vi "Autonomous Independent.vi"() -> ()   [LabVIEW 2014]
doc: "This VI is called when autonomous begins, and will automatically be terminated when autonomous ends. You can carry out timed or sensor driven robot movement independently without needing to return to the caller."
uses:
  <vilib>/Rock Robotics/Network Tables/SD Write Numeric Array.vi
  <vilib>/addons/control/pid/NI_PID_pid.lvlib
  <vilib>/addons/control/pid/pid.llb/PID (DBL).vi
  Robot Global Data.vi
  <vilib>/Rock Robotics/WPI/RobotDrive/WPI_RobotDriveMotorSelectorEnum.ctl
  <vilib>/Rock Robotics/WPI/CAN/TalonSRX/WPI_CANTalonSRX_APIControlMode.ctl
panel:
  in  "(Left) First Step":dbl
  in  "(Right) First Step":dbl
  in  "Left Wheel Distance":dbl
  in  "Right Wheel Distance":dbl
  in  "(Right) First Step":dbl
  in  "(Left) First Step":dbl
  # "Be sure to right-click and choose Data Operations>>Make Current Value default if you want to save the array values with the VI"
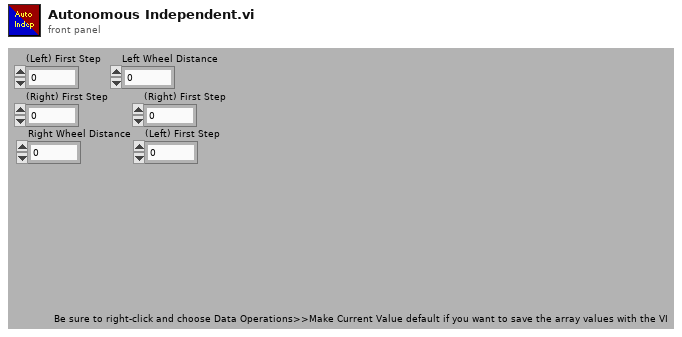
[diagram p1: front panel]
types:
  T1 = typedef "WPI_CANTalonSRX_APIControlMode.ctl" = enum8{"Percent VBus", "Speed", "Position", "Slave", "Unchanged / Invalid"}
  T2 = typedef "WPI_RobotDriveMotorSelectorEnum.ctl" = enum16{"Rear Left Motor", "Rear Right Motor", "Front Left Motor", "Front Right Motor"}
  T3 = typedef "WPI_JoystickDevRef.ctl" = cluster{"Device":T4}
  T4 = typedef "WPI_JoystickDeviceEnum.ctl" = enum16{"USB 0", "USB 1", "USB 2", "USB 3", "USB 4", "USB 5"}
  T5 = typedef "WPI_RobotDriveDevRef.ctl" = cluster{"DevStatus":errorcluster, "Motors[]":T6[], "Square Inputs":bool, "Max Output":dbl}
  T6 = typedef "WPI_MotorControlDeviceRef.ctl" = cluster{"DeviceStatus":errorcluster, "Type":T7, "PWM":cluster{"Controller":T8, "PWM Channel":T9, "DeadBand":T10}, "CAN":cluster{"Device Number":u8, "Control Mode":T11, "Semaphore":T12, "Max Vout":dbl, "TalonSRX Control Mode":T1}, "Invert":bool, "TransformRef":T13, "InvTransformRef":T13}
  T7 = typedef "WPI_MotorControlType.ctl" = enum16{"PWM", "CAN", "CANTalonSRX"}
  T8 = typedef "FPGA_TypedefDigitalModule.ctl" = enum16{"Controller 1"}
  T9 = typedef "FPGA_DIOPWMChannel.ctl" = enum8{"PWM 0", "PWM 1", "PWM 2", "PWM 3", "PWM 4", "PWM 5", "PWM 6", "PWM 7", "PWM 8", "PWM 9", "PWM MXP 0", "PWM MXP 1", "PWM MXP 2", "PWM MXP 3", "PWM MXP 4", "PWM MXP 5", "PWM MXP 6", "PWM MXP 7", "PWM MXP 8", "PWM MXP 9", "Invalid"}
  T10 = typedef "WPI_PWMDeadband.ctl" = cluster{"Name":string, "maxPositivePwm":i32, "minPositivePwm":i32, "centerPwm":i32, "maxNegativePwm":i32, "minNegativePwm":i32, "angularRange":u16}
  T11 = typedef "WPI_CANJaguar_ControlMode.ctl" = enum8{"Percent VBus", "Current", "Speed", "Position", "Voltage"}
  T12 = typedef "Semaphore RefNum" = refnum<k1>
  T13 = typedef "WPI_PWMTransform_ConPane.ctl" = refnum<vi>
  T14 = typedef "WPI_SwitchDevRef.ctl" = cluster{"DevStatus":errorcluster, "DIO Channel":T15, "Controller":T8, "CntIndex":T16, "Normally Closed":bool}
  T15 = typedef "FPGA_DIOChannel.ctl" = enum8{"DIO 0", "DIO 1", "DIO 2", "DIO 3", "DIO 4", "DIO 5", "DIO 6", "DIO 7", "DIO 8", "DIO 9", "DIO MXP 0", "DIO MXP 1", "DIO MXP 2", "DIO MXP 3", "DIO MXP 4", "DIO MXP 5", "DIO MXP 6", "DIO MXP 7", "DIO MXP 8", "DIO MXP 9", "DIO MXP 10", "DIO MXP 11", "DIO MXP 12", "DIO MXP 13", "DIO MXP 14", "DIO MXP 15", "Invalid"}
  T16 = typedef "FPGA_CounterCtrSystemIndex.ctl" = enum8{"Ctr 0", "Ctr 1", "Ctr 2", "Ctr 3", "Ctr 4", "Ctr 5", "Ctr 6", "Ctr 7", "Invalid"}
  T17 = typedef "WPI_CANTalonSRX_GlobalStatus.ctl" = cluster{"Applied Throttle":dbl, "Module Enabled":bool, "CAN Error":errorcluster, "Closed Loop Error":dbl, "Forward Limit Switch Closed":bool, "Reverse Limit Switch Closed":bool, "Sensor Position":dbl, "Sensor Velocity":dbl, "Current":dbl, "Sticky Fault - Over Temp":bool, "Sticky Fault - Under Voltage":bool, "Sticky Fault - Forward Limit":bool, "Sticky Fault - Reverse Limit":bool, "Sticky Fault - Forward Soft Limit":bool, "Sticky Fault - Reverse Soft Limit":bool, "Brake is Enabled":bool, "Encoder Position":dbl, "Encoder Velocity":dbl, "Encoder Index Count":dbl, "Encoder A Pin State":bool, "Encoder B Pin State":bool, "Encoder Index Pin State":bool, "Analog In":dbl, "Analog In Velocity":dbl, "Temperature (C)":dbl, "Battery Voltage":dbl}
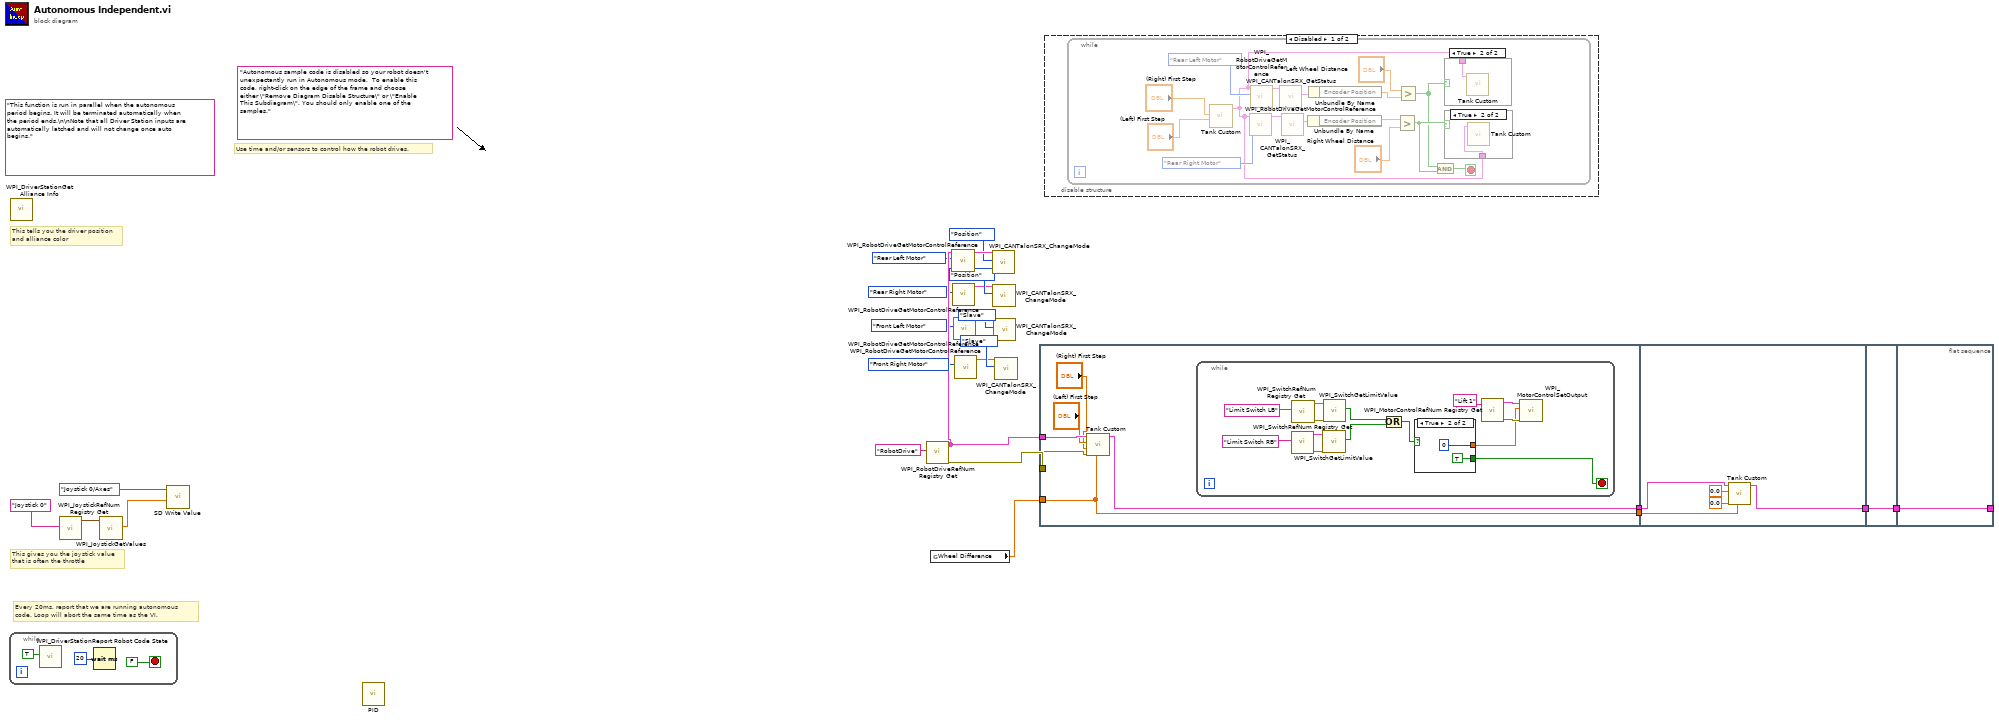
[diagram p0: block diagram]
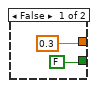
[diagram p5: hidden frame]
diagram:
  (unwired) "Autonomous sample code is disabled so your robot doesn't unexpectantly run in Autonomous mode.  To enable this code, right-click on the edge of the frame and choose either \"Remove Diagram Disable Structure\" or \"Enable This Subdiagram\". You should only enable one of the samples."
  (unwired) "This function is run in parallel when the autonomous period begins. It will be terminated automatically when the period ends.\n\nNote that all Driver Station inputs are automatically latched and will not change once auto begins."
  # "Every 20ms, report that we are running autonomous\ncode. Loop will abort the same time as the VI."
  # "This gives you the joystick value\nthat is often the throttle"
  # "Use time and/or sensors to control how the robot drives."
  # "This tells you the driver position\nand alliance color"
  n1 = while {
    stop <- FALSE stop-if-true
    n2 = call <vilib>:"WPI_DriverStationReport Robot Code State.vi"("Autonomous"=TRUE) -> ()  [unwired: 10 in, 1 out]
    n3 = Wait (ms)(milliseconds to wait=u32 20) -> ()  [unwired: 1 out]
  }
  n4 = call <vilib>:"WPI_DriverStationGet Alliance Info.vi"() -> ()  [unwired: 12 out]
  n5 = call <vilib>:"WPI_JoystickRefNum Registry Get.vi"("refnum name"="Joystick 0") -> ("JoystickDevRef"=w23:T3)  [unwired: 1 in, 9 out]
  n6 = call <vilib>:"WPI_JoystickGetValues.vi"("JoystickDevRef"=w23) -> ("Axes"=w21:dbl[])  [unwired: 6 in, 4 out]
  n7 = call-poly <vilib>:"SD Write Value.vi"("Numeric Array"=w21, "Name"="Joystick 0/Axes") -> ()  [unwired: 8 in, 2 out]
  n8 = call-poly <vilib>:"PID.vi"() -> ()  [unwired: 10 in, 2 out]
  n9 = call <vilib>:"WPI_RobotDriveRefNum Registry Get.vi"("refnum name"="RobotDrive") -> ("error out"=w15:errorcluster, "RobotDriveDevRef"=w12:T5)  [unwired: 1 in, 8 out]
  n10 = global read "Robot Global Data.vi" "Wheel Difference"() -> (w14:dbl)
  n11 = call <vilib>:"WPI_RobotDriveGetMotorControlReference.vi"("MotorIndex"=WPI_RobotDriveMotorSelectorEnum."Rear Left Motor", "RobotDriveDevRef"=w12) -> ("MotorControlDeviceRef"=w13:T6)  [unwired: 9 out]
  n12 = call <vilib>:"WPI_RobotDriveGetMotorControlReference.vi"("MotorIndex"=WPI_RobotDriveMotorSelectorEnum."Rear Right Motor") -> ("MotorControlDeviceRef"=w7:T6)  [unwired: 1 in, 9 out]
  n13 = call <vilib>:"WPI_RobotDriveGetMotorControlReference.vi"("MotorIndex"=WPI_RobotDriveMotorSelectorEnum."Front Left Motor") -> ("MotorControlDeviceRef"=w6:T6)  [unwired: 1 in, 9 out]
  n14 = call <vilib>:"WPI_RobotDriveGetMotorControlReference.vi"("MotorIndex"=WPI_RobotDriveMotorSelectorEnum."Front Right Motor") -> ("MotorControlDeviceRef"=w1:T6)  [unwired: 1 in, 9 out]
  n15 = call <vilib>:"WPI_CANTalonSRX_ChangeMode.vi"("Control Mode"=WPI_CANTalonSRX_APIControlMode."Position", "CAN Talon SRX Ref"=w13) -> ()  [unwired: 8 in, 2 out]
  n16 = call <vilib>:"WPI_CANTalonSRX_ChangeMode.vi"("Control Mode"=WPI_CANTalonSRX_APIControlMode."Position", "CAN Talon SRX Ref"=w7) -> ()  [unwired: 8 in, 2 out]
  n17 = call <vilib>:"WPI_CANTalonSRX_ChangeMode.vi"("Control Mode"=WPI_CANTalonSRX_APIControlMode."Slave", "CAN Talon SRX Ref"=w6) -> ()  [unwired: 8 in, 2 out]
  n18 = call <vilib>:"WPI_CANTalonSRX_ChangeMode.vi"("Control Mode"=WPI_CANTalonSRX_APIControlMode."Slave", "CAN Talon SRX Ref"=w1) -> ()  [unwired: 8 in, 2 out]
  n19 = flat-sequence {
    tunnel: w12 -> [w33]
    tunnel: w15 -> [w32]
    tunnel: [w31] -> w20
    tunnel: w14 -> [w30]
    tunnel: [w30] -> w19
    tunnel: [w53] -> w18
    tunnel: w20 -> [w54]
    tunnel: w19 -> [w52]
    tunnel: [w57] -> w17
    tunnel: w18 -> [w57]
    tunnel: [w58] -> _
    tunnel: w17 -> [w58]
    frame #0 {
      n20 = call <vilib>:"Tank Custom.vi"("Wheel Difference"=w30, "error in (no error)"=w32, "Right axis value"="(Right) First Step", "Left axis value"="(Left) First Step", "RobotDriveDevRef"=w33) -> ("RobotDriveDevRef"=w31:T5)  [unwired: 4 in, 2 out]
      n21 = while {
        stop <- w34 stop-if-true
        n22 = call <vilib>:"WPI_SwitchRefNum Registry Get.vi"("refnum name"="Limit Switch RB") -> ("error out"=w44:errorcluster, "SwitchDevRef"=w43:T14)  [unwired: 9 in]
        n23 = call <vilib>:"WPI_SwitchRefNum Registry Get.vi"("refnum name"="Limit Switch LB") -> ("error out"=w45:errorcluster, "SwitchDevRef"=w46:T14)  [unwired: 9 in]
        n24 = call <vilib>:"WPI_SwitchGetLimitValue.vi"("error in (no error)"=w44, "SwitchDevRef"=w43) -> ("Switch Pressed"=w40:bool)  [unwired: 7 in, 2 out]
        n25 = call <vilib>:"WPI_SwitchGetLimitValue.vi"("error in (no error)"=w45, "SwitchDevRef"=w46) -> ("Switch Pressed"=w41:bool)  [unwired: 7 in, 2 out]
        n26 = Or(x=w41, y=w40) -> (x .or. y?=w36:bool)
        n27 = case shown="True" w36 {
          tunnel: [0.3 0] -> w35
          tunnel: [FALSE TRUE] -> w34
          frame False {
          }
          frame True {
          }
        }
        n28 = call <vilib>:"WPI_MotorControlRefNum Registry Get.vi"("refnum name"="Lift 1") -> ("error out"=w39:errorcluster, "MotorControlDevRef"=w38:T6)  [unwired: 9 in]
        n29 = call <vilib>:"WPI_MotorControlSetOutput.vi"("error in (no error)"=w39, "Output"=w35, "MotorControlDevRef"=w38) -> ()  [unwired: 6 in, 3 out]
      }
    }
    frame #1 {
      n30 = call <vilib>:"Tank Custom.vi"("Wheel Difference"=w52, "Right axis value"=0.0, "Left axis value"=0.0, "RobotDriveDevRef"=w54) -> ("RobotDriveDevRef"=w53:T5)  [unwired: 5 in, 2 out]
    }
    frame #2 {
    }
    frame #3 {
    }
  }
  n31 = disable-structure shown="Disabled" {
    frame Disabled {
      n32 = while {
        stop <- w64 stop-if-true
        n33 = call <vilib>:"Tank Custom.vi"("Right axis value"="(Left) First Step", "Left axis value"="(Right) First Step") -> ("RobotDriveDevRef"=w61:T5)  [unwired: 7 in, 2 out]
        n34 = call <vilib>:"WPI_RobotDriveGetMotorControlReference.vi"("MotorIndex"=WPI_RobotDriveMotorSelectorEnum."Rear Right Motor", "RobotDriveDevRef"=w61) -> ("MotorControlDeviceRef"=w71:T6)  [unwired: 9 out]
        n35 = call <vilib>:"WPI_RobotDriveGetMotorControlReference.vi"("MotorIndex"=WPI_RobotDriveMotorSelectorEnum."Rear Left Motor", "RobotDriveDevRef"=w61) -> ("MotorControlDeviceRef"=w72:T6)  [unwired: 9 out]
        n36 = call <vilib>:"WPI_CANTalonSRX_GetStatus.vi"("CAN Talon SRX Ref"=w72) -> ("Talon SRX Status"=w69:T17)  [unwired: 8 in, 2 out]
        n37 = call <vilib>:"WPI_CANTalonSRX_GetStatus.vi"("CAN Talon SRX Ref"=w71) -> ("Talon SRX Status"=w70:T17)  [unwired: 8 in, 2 out]
        n38 = Unbundle By Name(w70) -> ("Encoder Position"=w68:dbl)
        n39 = Unbundle By Name(w69) -> ("Encoder Position"=w65:dbl)
        n40 = Greater?(x=w68, y="Right Wheel Distance") -> (0:w63:bool)
        n41 = Greater?(x="Left Wheel Distance", y=w65) -> (0:w62:bool)
        n42 = And(x=w62, y=w63) -> (x .and. y?=w64:bool)
        n43 = case shown="True" w62 {
          tunnel: w61 -> [_ w76]
          frame False {
          }
          frame True {
            n44 = call <vilib>:"Tank Custom.vi"("RobotDriveDevRef"=w76) -> ()  [unwired: 8 in, 3 out]
          }
        }
        n45 = case shown="True" w63 {
          tunnel: w61 -> [_ w75]
          frame False {
          }
          frame True {
            n46 = call <vilib>:"Tank Custom.vi"("RobotDriveDevRef"=w75) -> ()  [unwired: 8 in, 3 out]
          }
        }
      }
    }
    frame Enabled {
    }
  }
